vi "ER2007 Maintenance Panel.vi"() -> ()   [LabVIEW 2013]
uses:
  <vilib>/DAQmx/create/channels.llb/DAQmx Create Channel (DO-Digital Output).vi
  <vilib>/DAQmx/write.llb/DAQmx Write (Digital 1D Bool NChan 1Samp 1Line).vi
  Global ER2007.vi
  <vilib>/DAQmx/create/channels.llb/DAQmx Create Channel (DI-Digital Input).vi
  <vilib>/DAQmx/read.llb/DAQmx Read (Digital 1D Bool NChan 1Samp 1Line).vi
panel:
  out "Dev2Err":bool
  out "Lbl CJ1A":enum16{"CJ1A", "TC7B"}(ring)
  out "Lbl Pc1A":enum16{"Pc1A", "TC7A"}(ring)
  out "Lbl CJ1B":enum16{"CJ1B", "NOP8"}(ring)
  out "Lbl Pc1B":enum16{"Pc1B", "NOP7"}(ring)
  out "Lbl TC1B":enum16{"TC1B", "TC6B"}(ring)
  out "Lbl TC1A":enum16{"TC1A", "TC6A"}(ring)
  out "Lbl NOP1":enum16{"NOP1", "NOP6"}(ring)
  out "Ain 0-10":dbl format="%.3f"
  out "Ain 0-9":dbl format="%.3f"
  out "Ain 0-8":dbl format="%.3f"
  out "Ain 0-3":dbl format="%.3f"
  out "Ain 0-2":dbl format="%.3f"
  out "Ain 0-1":dbl format="%.3f"
  out "Ain 0-0":dbl format="%.3f"
  in  "Dout 1-0.11":bool
  in  "Dout 1-0.8":bool
  in  "Dout 1-0.13":bool
  out "Lbl PVol5":enum16{"PVol5", "PVol10"}(ring)
  out "Lbl PVol4":enum16{"PVol4", "PVol9"}(ring)
  out "Lbl PVol3":enum16{"PVol3", "PVol8"}(ring)
  out "Lbl PVol2":enum16{"PVol2", "PVol7"}(ring)
  out "Lbl PVol1":enum16{"PVol1", "PVol6"}(ring)
  out "Lbl Pdp5":enum16{"Pdp5", "Pdp10"}(ring)
  out "Lbl Pdp4":enum16{"Pdp4", "Pdp9"}(ring)
  out "Lbl Pdp3":enum16{"Pdp3", "Pdp8"}(ring)
  out "Lbl Pdp2":enum16{"Pdp2", "Pdp7"}(ring)
  out "Lbl Pdp1":enum16{"Pdp1", "Pdp6"}(ring)
  out "Lbl CJ5B":enum16{"CJ5B", "Pc10"}(ring)
  out "Lbl NOP5":enum16{"NOP5", "Pc9"}(ring)
  out "Lbl CJ3B":enum16{"CJ3B", "Pc8"}(ring)
  out "Lbl NOP3":enum16{"NOP3", "Pc7"}(ring)
  out "Lbl Pc2A":enum16{"Pc2A", "Pc6"}(ring)
  out "Lbl CJ5A":enum16{"CJ5A", "CJ9B"}(ring)
  out "Lbl Pc5B":enum16{"Pc5B", "CJ9A"}(ring)
  out "Lbl CJ4B":enum16{"CJ4B", "CJ8B"}(ring)
  out "Lbl CJ4A":enum16{"CJ4A", "CJ8A"}(ring)
  out "Lbl CJ3A":enum16{"CJ3A", "CJ7B"}(ring)
  out "Lbl Pc3B":enum16{"Pc3B", "CJ7A"}(ring)
  out "Lbl CJ2B":enum16{"CJ2B", "CJ6B"}(ring)
  out "Lbl CJ2A":enum16{"CJ2A", "CJ6A"}(ring)
  out "Lbl Pc4A":enum16{"Pc4A", "TC10B"}(ring)
  out "Lbl TC5B":enum16{"TC5B", "TC10A"}(ring)
  out "Lbl Pc5A":enum16{"Pc5A", "TC9B"}(ring)
  out "Lbl Pc4B":enum16{"Pc4B", "TC9A"}(ring)
  out "Lbl TC4A":enum16{"TC4A", "TC8B"}(ring)
  out "Lbl NOP4":enum16{"NOP4", "TC8A"}(ring)
  out "Lbl TC3A":enum16{"TC3A", "TC7B"}(ring)
  out "Lbl Pc3A":enum16{"Pc3A", "TC7A"}(ring)
  out "Lbl TC5A":enum16{"TC5A", "NOP10"}(ring)
  out "Lbl TC4B":enum16{"TC4B", "NOP9"}(ring)
  out "Lbl TC3B":enum16{"TC3B", "NOP8"}(ring)
  out "Lbl Pc2B":enum16{"Pc2B", "NOP7"}(ring)
  out "Lbl TC2B":enum16{"TC2B", "TC6B"}(ring)
  out "Lbl TC2A":enum16{"TC2A", "TC6A"}(ring)
  out "Lbl NOP2":enum16{"NOP2", "NOP6"}(ring)
  out "Ain 1-31":dbl format="%.3f"
  out "Ain 1-30":dbl format="%.3f"
  out "Ain 1-15":dbl format="%.3f"
  out "Ain 1-14":dbl format="%.3f"
  in  "Dout 1-0.3":bool
  in  "Dout 1-0.0":bool
  out "P0-2.1":bool caption="P2.1 - Busy 2"
  out "P0-2.0":bool caption="P2.0 - Busy 1"
  in  "Dout 0-1.6":bool
  out "Err 6":bool
  out "Err 5":bool
  out "NAII Time":u32
  out "NAII Err":i32
  in  "Wait (ms)":u32=1500
  out "Freq":dbl
  in  "Set":bool
  out "Err 3":bool
  out "Err 4":bool
  out "Exec Time":u32
  out "Signal":dbl format="%.4f"
  out "Phase":dbl format="%.3f"
  out "Reference":dbl format="%.4f"
  in  "Update":bool
  in  "Gen Off/On":bool
  in  "Ampl (Vrms)":dbl=1.0 min=0.1 max=10.0 format="%.2f"
  in  "Freq (Hz)":dbl=1000.0 min=20.0 max=100000.0
  out "Net 4-1":dbl format="%.3f"
  out "Net 4-0":dbl format="%.3f"
  out "Net 3-1":dbl format="%.3f"
  out "Net 3-0":dbl format="%.3f"
  out "Net 2-1":dbl format="%.3f"
  out "Net 2-0":dbl format="%.3f"
  out "Net 1-1":dbl format="%.3f"
  out "Net 1-0":dbl format="%.3f"
  out "Net 0-1":dbl format="%.3f"
  out "Net 0-0":dbl format="%.3f"
  in  "EUs 1":bool
  out "Ain 1-29":dbl format="%.3f"
  out "Ain 1-27":dbl format="%.3f"
  out "Ain 1-26":dbl format="%.3f"
  out "Ain 1-25":dbl format="%.3f"
  out "Ain 1-24":dbl format="%.3f"
  out "Ain 1-23":dbl format="%.3f"
  out "Ain 1-22":dbl format="%.3f"
  out "Ain 1-21":dbl format="%.3f"
  out "Ain 1-19":dbl format="%.3f"
  out "Ain 1-18":dbl format="%.3f"
  out "Ain 1-17":dbl format="%.3f"
  out "Ain 1-16":dbl format="%.3f"
  in  "EUs 0":bool
  out "Ain 1-13":dbl format="%.3f"
  out "Ain 1-11":dbl format="%.3f"
  out "Ain 1-10":dbl format="%.3f"
  out "Ain 1-9":dbl format="%.3f"
  out "Ain 1-8":dbl format="%.3f"
  out "Ain 1-7":dbl format="%.3f"
  out "Ain 1-6":dbl format="%.3f"
  out "Ain 1-5":dbl format="%.3f"
  out "Ain 1-3":dbl format="%.3f"
  out "Ain 1-2":dbl format="%.3f"
  out "Ain 1-1":dbl format="%.3f"
  out "Ain 1-0":dbl format="%.3f"
  out "Err 7":bool
  in  "AllOff 0":bool
  in  "Dout 0-1.4":bool
  in  "Dout 0-1.3":bool
  in  "Dout 0-1.2":bool
  in  "Dout 0-1.1":bool
  in  "Dout 0-1.0":bool
  in  "Dout 0-0.7":bool
  in  "Dout 1-0.5":bool
  in  "Dout 0-0.5":bool
  in  "Dout 0-0.4":bool
  in  "Dout 0-0.3":bool
  out "Dev1Err":bool
  in  "Dout 0-0.2":bool
  in  "Dout 0-0.1":bool
  in  "Dout 0-0.0":bool
  in  "Exit":bool
  # "ER2007 Maintenance Panel"
  # "Galil CDS-3310"
  # "Dev1 PCI-6220 Douts"
  # "Dev1 PCI-6220 Ains"
  # "Dev2 PCI-6224 Analog Ins"
  # "GPIB0 - Signal Gen"
  # "Error"
  # "Dev2 PCI-6224 Douts"
  # "PCI-6224 Dins"
  # "Error"
  # "GPIB1 - Volts/Phase"
  # "Error"
  # "Error"
  # "Error"
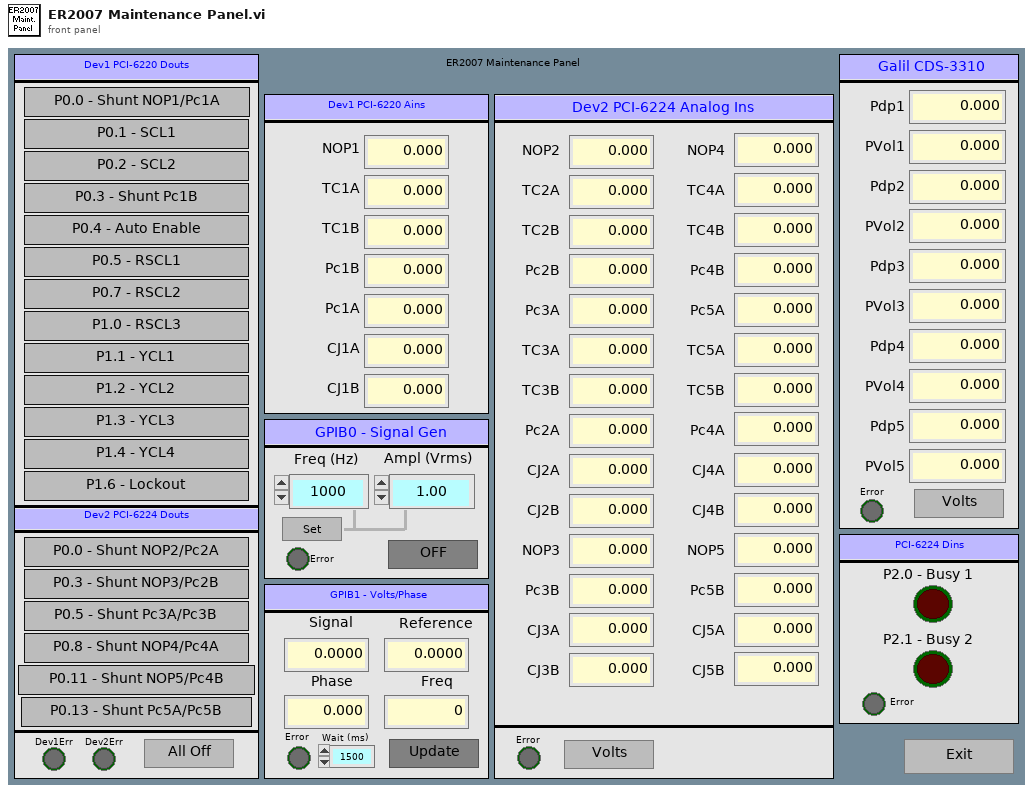
[diagram p1: front panel]
types:
  T1 = enum16{"TOTAL", "FUNDAMENTAL", "IN PHASE", "QUADRATURE", "PHASE ANGLE", "THD"}
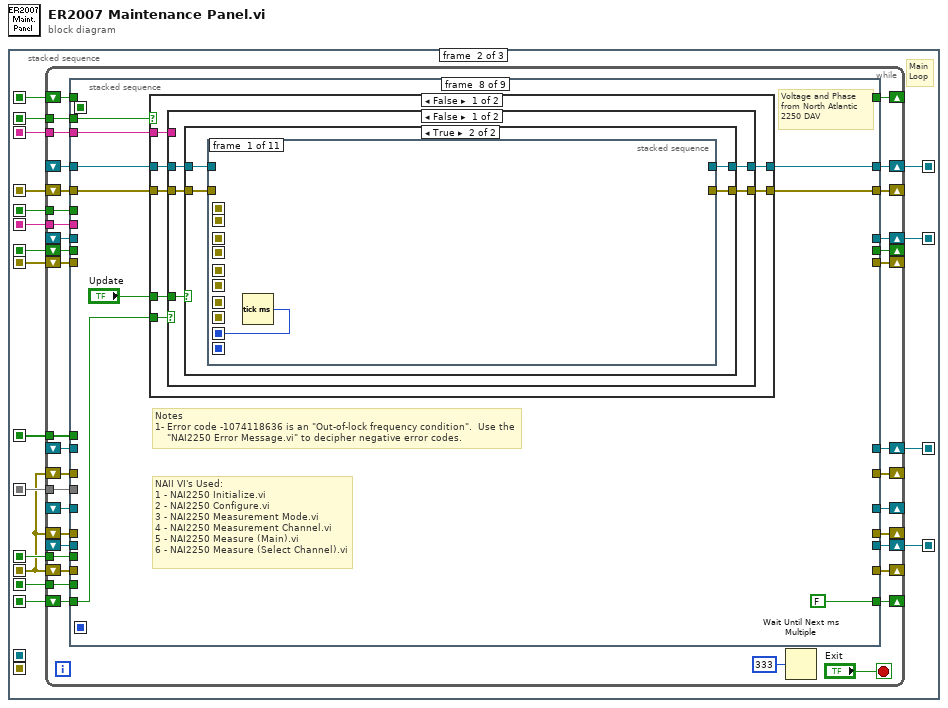
[diagram p0: block diagram]
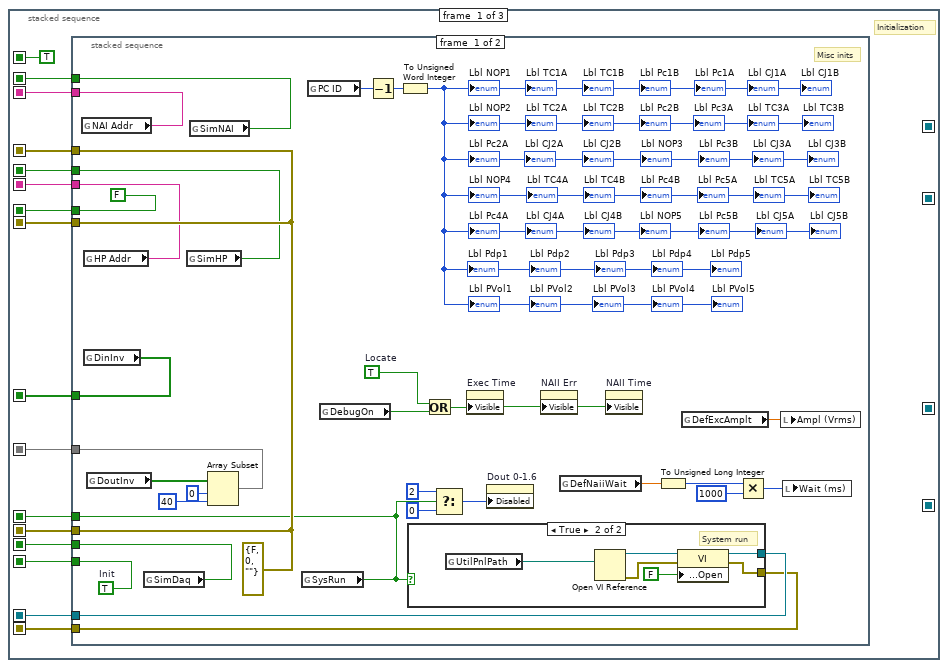
[diagram p2: hidden frame]
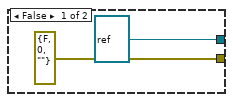
[diagram p3: hidden frame]
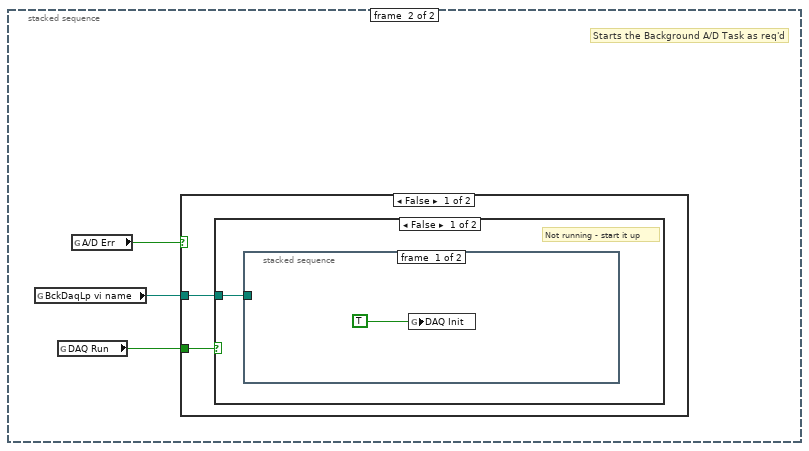
[diagram p4: hidden frame]
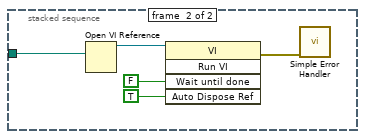
[diagram p5: hidden frame]
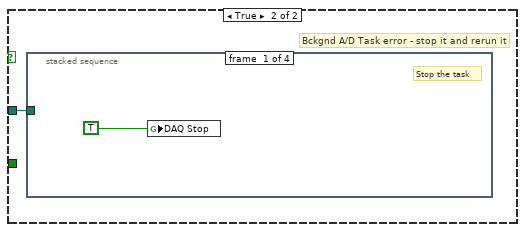
[diagram p7: hidden frame]
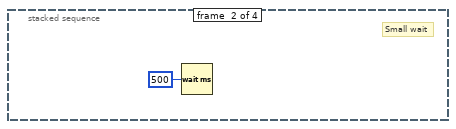
[diagram p8: hidden frame]
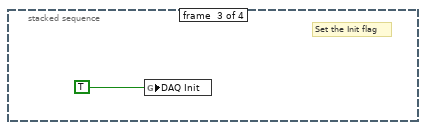
[diagram p9: hidden frame]
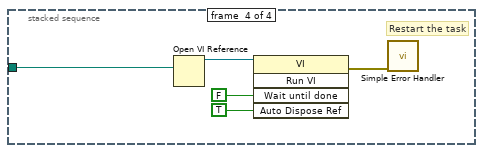
[diagram p10: hidden frame]
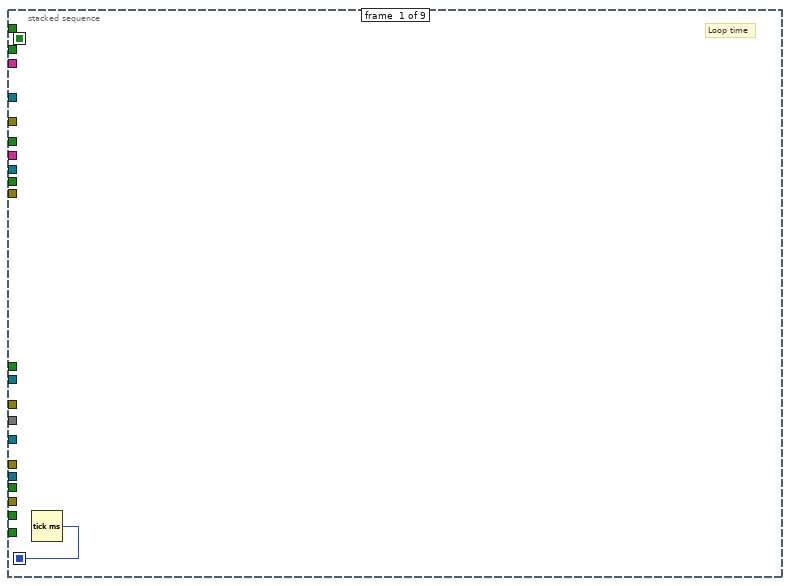
[diagram p11: hidden frame]
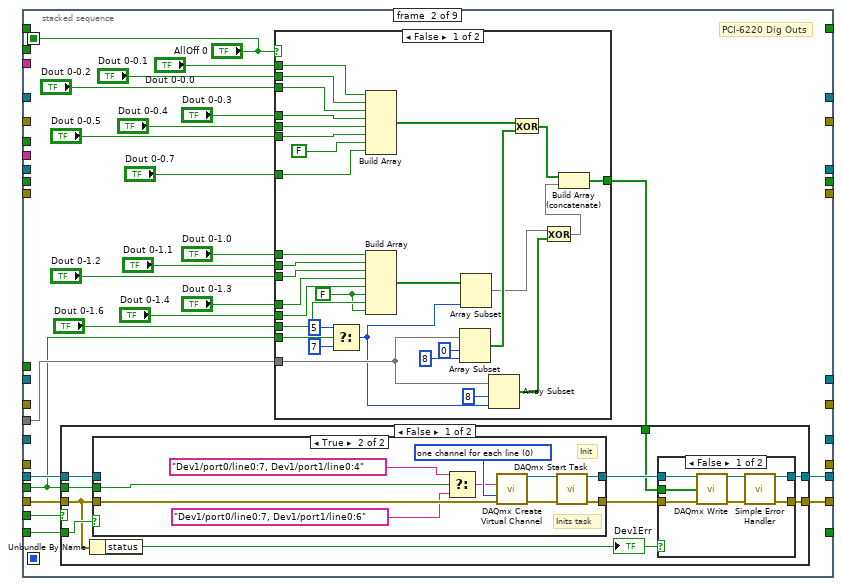
[diagram p12: hidden frame]
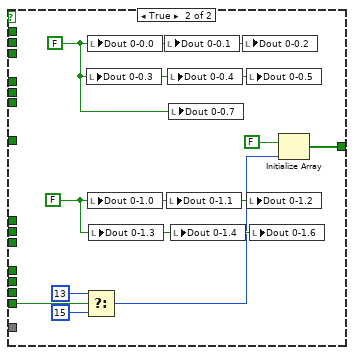
[diagram p16: hidden frame]
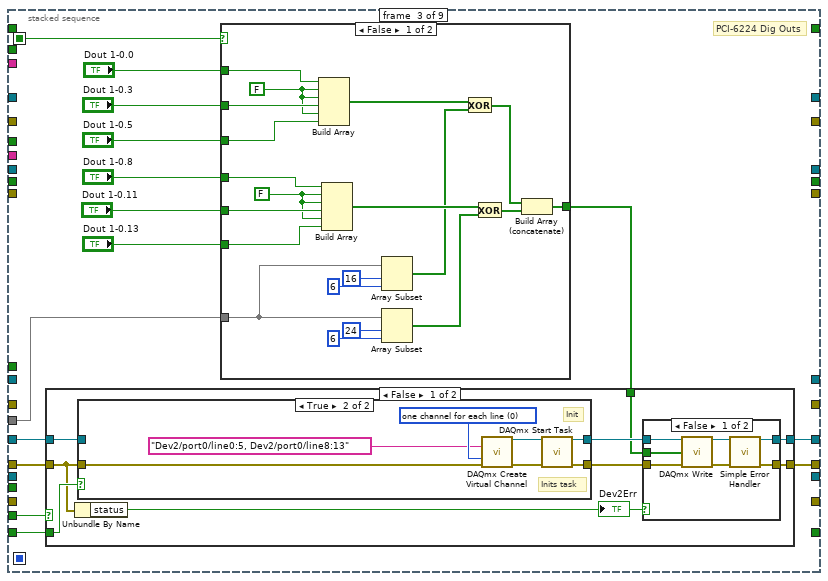
[diagram p17: hidden frame]
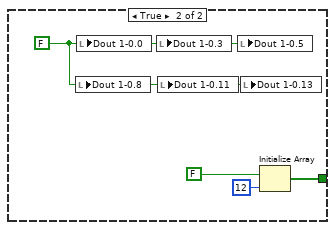
[diagram p18: hidden frame]
diagram:
  n1 = stacked-sequence {
    seq-local: [w16 _ _] -> [_ w91 _]
    seq-local: [w15 _ _] -> [_ w93 _]
    seq-local: [w14 _ _] -> [_ w76 _]
    seq-local: [w13 _ _] -> [_ w92 w633]
    seq-local: [w12 _ _] -> [_ w78 w638]
    seq-local: [w11 _ _] -> [_ _ w640]
    seq-local: [w10 _ _] -> [_ _ w639]
    seq-local: [_ w90 _] -> [_ _ w637]
    seq-local: [_ w89 _] -> [_ _ w636]
    seq-local: [w9 _ _] -> [_ w88 w632]
    seq-local: [w8 _ _] -> [_ w86 _]
    seq-local: [w7 _ _] -> [_ w87 _]
    seq-local: [w6 _ _] -> [_ w85 w631]
    seq-local: [w5 _ _] -> [_ w84 _]
    seq-local: [w4 _ _] -> [_ w83 _]
    seq-local: [w3 _ _] -> [_ w82 _]
    seq-local: [_ w81 _] -> [_ _ w635]
    seq-local: [_ w80 _] -> [_ _ w634]
    seq-local: [w2 _ _] -> [_ w79 _]
    seq-local: [TRUE _ _] -> [_ w77 _]
    frame #0 {
      # "Initialization"
      n2 = stacked-sequence {
        tunnel: [w29 _] -> w16
        tunnel: [w46 _] -> w15
        tunnel: [w43 _] -> w14
        tunnel: [w35 _] -> w13
        tunnel: [w25 _] -> w12
        tunnel: [w45 _] -> w11
        tunnel: [w44 _] -> w10
        tunnel: [w41 _] -> w9
        tunnel: [w40 _] -> w8
        tunnel: [w43 _] -> w7
        tunnel: [w38 _] -> w6
        tunnel: [w39 _] -> w5
        tunnel: [w43 _] -> w4
        tunnel: [FALSE _] -> w3
        tunnel: [w34 _] -> w2
        frame #0 {
          w26 = TRUE  # Locate
          w43 = errorcluster {"status"=FALSE, "code"=0, "source"=""} ("error out")
          w46 = TRUE  # Init
          # "Misc inits"
          n3 = global read "Global ER2007.vi" "NAI Addr"() -> (w40:string)
          n4 = global read "Global ER2007.vi" "HP Addr"() -> (w39:string)
          n5 = global read "Global ER2007.vi" "DinInv"() -> (w34:bool[])
          n6 = global read "Global ER2007.vi" "DoutInv"() -> (w30:bool[])
          n7 = global read "Global ER2007.vi" "SimDaq"() -> (w35:bool)
          n8 = global read "Global ER2007.vi" "SimHP"() -> (w38:bool)
          n9 = global read "Global ER2007.vi" "SimNAI"() -> (w41:bool)
          n10 = Array Subset(array=w30, index=0, length=40) -> (w29:bool[])
          n11 = global read "Global ER2007.vi" "SysRun"() -> (w25:bool)
          n12 = global read "Global ER2007.vi" "PC ID"() -> (w21:i32)
          n13 = global read "Global ER2007.vi" "DebugOn"() -> (w28:bool)
          n14 = Decrement(x=w21) -> (x-1=w20:i32)
          n15 = To Unsigned Word Integer(number=w20) -> (unsigned 16bit integer=→"Lbl NOP2" →"Lbl TC2A" →"Lbl Pc2A" →"Lbl TC4B" →"Lbl TC5A" →"Lbl CJ5B" →"Lbl NOP5" →"Lbl CJ3B" →"Lbl CJ5A" →"Lbl Pc4A" →"Lbl Pc5A" →"Lbl Pc2B" →"Lbl TC3B" →"Lbl TC3A" →"Lbl TC4A" →"Lbl CJ2B" →"Lbl CJ3A" →"Lbl CJ4B" →"Lbl NOP3" →"Lbl CJ4A" →"Lbl CJ2A" →"Lbl Pc3A" →"Lbl NOP4" →"Lbl Pc3B" →"Lbl Pc4B" →"Lbl Pc5B" →"Lbl TC2B" →"Lbl TC5B" →"Lbl Pdp1" →"Lbl Pdp2" →"Lbl Pdp3" →"Lbl Pdp4" →"Lbl Pdp5" →"Lbl PVol1" →"Lbl PVol2" →"Lbl PVol3" →"Lbl PVol4" →"Lbl PVol5" →"Lbl NOP1" →"Lbl TC1A" →"Lbl TC1B" →"Lbl Pc1B" →"Lbl Pc1A" →"Lbl CJ1A" →"Lbl CJ1B":u16)
          n16 = case shown="True" w25 {
            tunnel: [refnum<vi> refnum w51] -> w45
            tunnel: [errorcluster {"status"=FALSE, "code"=0, "source"=""} ("error out") w50] -> w44
            frame False {
            }
            frame True {
              # "System run"
              n17 = global read "Global ER2007.vi" "UtilPnlPath"() -> (w49:path)
              n18 = Open VI Reference(vi path=w49) -> (vi reference=w54:refnum<vi>, error out=w53:errorcluster)  [unwired: 5 in]
              n19 = property class="VI"(reference=w54, error in=w53, "Front Panel Window:Open"=FALSE) -> (reference out=w51:refnum<vi>, error out=w50:errorcluster)
            }
          }
          n20 = Or(x=w26, y=w28) -> (x .or. y?=w27:bool)
          n21 = Select(t=u8 2, s=w25, f=u8 0 ("Disabled")) -> (s? t:f=w24:u8)
          n22 = property on="Exec Time" class="DigNum (strict)"("Visible"=w27) -> ()  [unwired: 2 in, 2 out]
          n23 = property on="Dout 0-1.6" class="Bool (strict)"("Disabled"=w24) -> ()  [unwired: 2 in, 2 out]
          n24 = property on="NAII Err" class="DigNum (strict)"("Visible"=w27) -> ()  [unwired: 2 in, 2 out]
          n25 = global read "Global ER2007.vi" "DefNaiiWait"() -> (w36:dbl)
          n26 = property on="NAII Time" class="DigNum (strict)"("Visible"=w27) -> ()  [unwired: 2 in, 2 out]
          n27 = To Unsigned Long Integer(number=w36) -> (unsigned 32bit integer=w33:u32)
          n28 = global read "Global ER2007.vi" "DefExcAmplt"() -> (w37:dbl)
          n29 = Multiply(x=w33, y=u32 1000) -> (x*y=w18:u32)
          n30 = local write "Ampl (Vrms)"(w37) -> ()
          n31 = local write "Wait (ms)"(w18) -> ()
        }
        frame #1 {
          # "Starts the Background A/D Task as req'd"
          n32 = global read "Global ER2007.vi" "BckDaqLp vi name"() -> (w56:path)
          n33 = global read "Global ER2007.vi" "DAQ Run"() -> (w55:bool)
          n34 = global read "Global ER2007.vi" "A/D Err"() -> (w57:bool)
          n35 = case shown="False" w57 {
            tunnel: w55 -> [w59 _]
            tunnel: w56 -> [w58 w67]
            frame False {
              n36 = case shown="False" w59 {
                tunnel: w58 -> [w60 _]
                frame False {
                  # "Not running - start it up"
                  n37 = stacked-sequence {
                    tunnel: w60 -> [_ w62]
                    frame #0 {
                      n38 = global write "Global ER2007.vi" "DAQ Init"(TRUE ("A/D Init")) -> ()
                    }
                    frame #1 {
                      n39 = Open VI Reference(vi path=w62) -> (vi reference=w66:refnum<vi>)  [unwired: 5 in, 1 out]
                      n40 = invoke class="VI" method="Run VI"(reference=w66, "Wait until done"=FALSE, "Auto Dispose Ref"=TRUE) -> (error out=w63:errorcluster)  [unwired: 2 in, 4 out]
                      n41 = call <vilib>:"Simple Error Handler.vi"("error in (no error)"=w63) -> ()  [unwired: 4 in, 5 out]
                    }
                  }
                }
                frame True {
                  # "The bckgnd task is already\nrunning - do nothing"
                }
              }
            }
            frame True {
              # "Bckgnd A/D Task error - stop it and rerun it"
              n42 = stacked-sequence {
                tunnel: w67 -> [_ _ _ w71]
                frame #0 {
                  # "Stop the task"
                  n43 = global write "Global ER2007.vi" "DAQ Stop"(TRUE ("A/D Stop")) -> ()
                }
                frame #1 {
                  # "Small wait"
                  n44 = Wait (ms)(milliseconds to wait=u32 500) -> ()  [unwired: 1 out]
                }
                frame #2 {
                  # "Set the Init flag"
                  n45 = global write "Global ER2007.vi" "DAQ Init"(TRUE ("A/D Init")) -> ()
                }
                frame #3 {
                  # "Restart the task"
                  n46 = Open VI Reference(vi path=w71) -> (vi reference=w75:refnum<vi>)  [unwired: 5 in, 1 out]
                  n47 = invoke class="VI" method="Run VI"(reference=w75, "Wait until done"=FALSE, "Auto Dispose Ref"=TRUE) -> (error out=w72:errorcluster)  [unwired: 2 in, 4 out]
                  n48 = call <vilib>:"Simple Error Handler.vi"("error in (no error)"=w72) -> ()  [unwired: 4 in, 5 out]
                }
              }
            }
          }
        }
      }
    }
    frame #1 {
      # "Main\nLoop"
      n49 = while {
        shift-right: [w127] -> _
        shift-left: w93 -> [w126]
        shift-right: [w124] -> _
        shift-left: w76 -> [w125]
        shift-right: [w123] -> w90
        shift-left: _ -> [w122]
        tunnel: w92 -> [w121]
        tunnel: w91 -> [w120]
        shift-right: [w116] -> _
        shift-left: w76 -> [w119]
        shift-right: [w117] -> w89
        shift-left: _ -> [w118]
        tunnel: w88 -> [w115]
        shift-right: [w113] -> _
        shift-left: w87 -> [w114]
        tunnel: w86 -> [w112]
        shift-right: [w111] -> w80
        shift-left: _ -> [w110]
        tunnel: w85 -> [w109]
        tunnel: w84 -> [w108]
        shift-right: [w106] -> _
        shift-left: w83 -> [w107]
        shift-right: [w105] -> w81
        shift-left: _ -> [w104]
        shift-right: [w102] -> _
        shift-left: w82 -> [w103]
        tunnel: w79 -> [w101]
        tunnel: w78 -> [w100]
        shift-right: [w99] -> _
        shift-left: w77 -> [w98]
        shift-right: [w95] -> _
        shift-left: _ -> [w96]
        shift-right: [w94] -> _
        shift-left: w76 -> [w97]
        stop <- "Exit" stop-if-true
        n50 = stacked-sequence {
          seq-local: [w130 _ _ _ _ _ _ _ _] -> [_ _ _ _ _ _ _ _ w629]
          seq-local: [_ "AllOff 0" _ _ _ _ _ _ _] -> [_ _ w233 _ _ _ _ _ _]
          tunnel: [_ _ _ _ _ _ _ FALSE _] -> w127
          tunnel: w126 -> [_ w153 w235 w304 _ _ w427 w485 _]
          tunnel: w125 -> [_ w152 _ _ _ _ _ _ _]
          tunnel: [_ w151 _ _ _ _ _ _ _] -> w124
          tunnel: [_ w150 _ _ _ _ _ _ _] -> w123
          tunnel: w122 -> [_ w149 _ _ _ _ _ _ _]
          tunnel: w121 -> [_ w135 w234 w305 _ _ _ _ _]
          tunnel: w120 -> [_ w134 w225 _ _ _ _ _ _]
          tunnel: w119 -> [_ _ _ w303 _ _ _ _ _]
          tunnel: w118 -> [_ _ _ w302 _ _ _ _ _]
          tunnel: [_ _ _ w301 _ _ _ _ _] -> w117
          tunnel: [_ _ _ w300 _ _ _ _ _] -> w116
          tunnel: w115 -> [_ _ _ _ _ _ _ w488 _]
          tunnel: w114 -> [_ _ _ _ _ _ _ w487 _]
          tunnel: [_ _ _ _ _ _ _ w486 _] -> w113
          tunnel: w112 -> [_ _ _ _ _ _ _ w484 _]
          tunnel: [_ _ _ _ _ _ _ w483 _] -> w111
          tunnel: w110 -> [_ _ _ _ _ _ _ w482 _]
          tunnel: w109 -> [_ _ _ _ _ _ w429 _ _]
          tunnel: w108 -> [_ _ _ _ _ _ w428 _ _]
          tunnel: w107 -> [_ _ _ _ _ _ w426 _ _]
          tunnel: [_ _ _ _ _ _ w425 _ _] -> w106
          tunnel: [_ _ _ _ _ _ w424 _ _] -> w105
          tunnel: w104 -> [_ _ _ _ _ _ w423 _ _]
          tunnel: w103 -> [_ _ _ _ _ _ w422 _ _]
          tunnel: [_ _ _ _ _ _ w421 _ _] -> w102
          tunnel: w101 -> [_ _ _ w294 _ _ _ _ _]
          tunnel: w100 -> [_ w132 _ w293 _ _ _ _ _]
          tunnel: [_ _ _ _ "EUs 0" _ _ _ _] -> w99
          tunnel: w98 -> [_ _ _ _ w388 _ _ _ _]
          tunnel: w97 -> [_ _ w239 _ _ _ _ _ _]
          tunnel: w96 -> [_ _ w238 _ _ _ _ _ _]
          tunnel: [_ _ w237 _ _ _ _ _ _] -> w95
          tunnel: [_ _ w236 _ _ _ _ _ _] -> w94
          frame #0 {
            # "Loop time"
            n51 = Tick Count (ms)() -> (millisecond timer value=w130:u32)
          }
          frame #1 {
            # "PCI-6220 Dig Outs"
            n52 = case shown="False" "AllOff 0" {
              tunnel: "Dout 0-0.0" -> [w216 _]
              tunnel: "Dout 0-0.1" -> [w215 _]
              tunnel: "Dout 0-0.2" -> [w214 _]
              tunnel: "Dout 0-0.3" -> [w213 _]
              tunnel: "Dout 0-0.4" -> [w212 _]
              tunnel: "Dout 0-0.5" -> [w211 _]
              tunnel: "Dout 0-0.7" -> [w210 _]
              tunnel: "Dout 0-1.0" -> [w203 _]
              tunnel: "Dout 0-1.1" -> [w204 _]
              tunnel: "Dout 0-1.2" -> [w205 _]
              tunnel: "Dout 0-1.3" -> [w202 _]
              tunnel: "Dout 0-1.4" -> [w201 _]
              tunnel: [w198 w223] -> w136
              tunnel: w134 -> [w195 _]
              tunnel: "Dout 0-1.6" -> [w197 _]
              tunnel: w132 -> [w188 w220]
              frame False {
                w196 = FALSE ("element")
                n53 = Select(t=5 ("length"), s=w188, f=7) -> (s? t:f=w187:i32)
                n54 = Build Array(w216, w215, w214, w213, w212, w211, FALSE ("element"), w210) -> (w209:bool[])
                n55 = Build Array(w203, w204, w205, w202, w201, w196, w197, w196) -> (w194:bool[])
                n56 = Array Subset(array=w195, index=0, length=8) -> (w206:bool[])
                n57 = Array Subset(array=w194, length=w187) -> (w193:bool[])  [unwired: 1 in]
                n58 = Array Subset(array=w195, index=8, length=w187) -> (w200:bool[])
                n59 = Exclusive Or(1:w206, 2:w209) -> (0:w199:bool[])
                n60 = Exclusive Or(1:w200, 2:w193) -> (0:w191:bool[])
                n61 = Build Array (concatenate)(w199, w191) -> (w198:bool[])
              }
              frame True {
                w221 = FALSE ("Dout 0-1.0")
                w222 = FALSE ("Dout 0-0.1")
                n62 = Select(t=13 ("dimension size"), s=w220, f=15 ("dimension size")) -> (s? t:f=w217:i32)
                n63 = local write "Dout 0-0.3"(w222) -> ()
                n64 = local write "Dout 0-0.0"(w222) -> ()
                n65 = local write "Dout 0-1.0"(w221) -> ()
                n66 = local write "Dout 0-1.3"(w221) -> ()
                n67 = local write "Dout 0-0.1"(w222) -> ()
                n68 = local write "Dout 0-1.1"(w221) -> ()
                n69 = local write "Dout 0-0.4"(w222) -> ()
                n70 = local write "Dout 0-0.7"(w222) -> ()
                n71 = local write "Dout 0-1.4"(w221) -> ()
                n72 = local write "Dout 0-0.2"(w222) -> ()
                n73 = local write "Dout 0-0.5"(w222) -> ()
                n74 = local write "Dout 0-1.2"(w221) -> ()
                n75 = local write "Dout 0-1.6"(w221) -> ()
                n76 = Initialize Array(FALSE, w217) -> (w223:bool[])
              }
            }
            n77 = case shown="False" w135 {
              tunnel: w153 -> [w163 _]
              tunnel: w152 -> [w156 w184]
              tunnel: [w161 w184] -> w151
              tunnel: [w160 w185] -> w150
              tunnel: w149 -> [w158 w185]
              tunnel: w136 -> [w157 _]
              tunnel: w132 -> [w154 _]
              frame False {
                n78 = Unbundle By Name(w156) -> ("status"=w155:bool)
                "Dev1Err" <- w155
                n79 = case shown="True" w163 {
                  tunnel: w156 -> [w172 w181]
                  tunnel: [w173 w180] -> w162
                  tunnel: [w172 w179] -> w159
                  tunnel: w158 -> [w173 _]
                  tunnel: w154 -> [_ w174]
                  frame False {
                  }
                  frame True {
                    w178 = 0 items=["one channel for each line", "one channel for all lines"] ("line grouping")
                    # "Init"
                    # "Inits task"
                    n80 = Select(t=tag "Dev1/port0/line0:7, Dev1/port1/line0:4" ("lines"), s=w174, f=tag "Dev1/port0/line0:7, Dev1/port1/line0:6" ("lines")) -> (s? t:f=w177:tag)
                    n81 = call-poly <vilib>:"DAQmx Create Virtual Channel.vi"("lines"=w177, "line grouping"=w178, "error in"=w181) -> ("task out"=w183:refnum<k21>, "error out"=w182:errorcluster)  [unwired: 11 in]
                    n82 = call <vilib>:"DAQmx Start Task.vi"("task/channels in"=w183, "error in"=w182) -> ("task out"=w180:refnum<k21>, "error out"=w179:errorcluster)  [unwired: 12 in]
                  }
                }
                n83 = case shown="False" w155 {
                  tunnel: w159 -> [w169 w170]
                  tunnel: w162 -> [w168 w171]
                  tunnel: [w165 w170] -> w161
                  tunnel: [w167 w171] -> w160
                  tunnel: w157 -> [w164 _]
                  frame False {
                    n84 = call-poly <vilib>:"DAQmx Write.vi"("task/channels in"=w168, "data"=w164, "error in"=w169) -> ("task out"=w167:refnum<k21>, "error out"=w166:errorcluster)  [unwired: 10 in, 1 out]
                    n85 = call <vilib>:"Simple Error Handler.vi"("error in (no error)"=w166) -> ("error out"=w165:errorcluster)  [unwired: 4 in, 4 out]
                  }
                  frame True {
                    # "Prev error"
                  }
                }
              }
              frame True {
                # "Simulation"
              }
            }
          }
          frame #2 {
            # "PCI-6224 Dig Outs"
            n86 = case shown="False" w233 {
              tunnel: "Dout 1-0.3" -> [w259 _]
              tunnel: "Dout 1-0.0" -> [w258 _]
              tunnel: "Dout 1-0.5" -> [w257 _]
              tunnel: "Dout 1-0.11" -> [w255 _]
              tunnel: "Dout 1-0.8" -> [w254 _]
              tunnel: "Dout 1-0.13" -> [w253 _]
              tunnel: [w251 w261] -> w226
              tunnel: w225 -> [w241 _]
              frame False {
                w252 = FALSE ("element")
                w256 = FALSE ("element")
                n87 = Build Array(w258, w256, w256, w259, w256, w257) -> (w250:bool[])
                n88 = Build Array(w254, w252, w252, w255, w252, w253) -> (w249:bool[])
                n89 = Array Subset(array=w241, index=16, length=6) -> (w244:bool[])
                n90 = Array Subset(array=w241, index=24, length=6) -> (w240:bool[])
                n91 = Exclusive Or(1:w244, 2:w250) -> (0:w247:bool[])
                n92 = Exclusive Or(1:w240, 2:w249) -> (0:w248:bool[])
                n93 = Build Array (concatenate)(w247, w248) -> (w251:bool[])
              }
              frame True {
                w263 = FALSE
                n94 = local write "Dout 1-0.8"(w263) -> ()
                n95 = local write "Dout 1-0.0"(w263) -> ()
                n96 = local write "Dout 1-0.3"(w263) -> ()
                n97 = local write "Dout 1-0.11"(w263) -> ()
                n98 = local write "Dout 1-0.5"(w263) -> ()
                n99 = local write "Dout 1-0.13"(w263) -> ()
                n100 = Initialize Array(FALSE, 12 ("dimension size")) -> (w261:bool[])
              }
            }
            n101 = case shown="False" w234 {
              tunnel: w235 -> [w272 _]
              tunnel: w239 -> [w265 w290]
              tunnel: [w270 w290] -> w236
              tunnel: [w269 w291] -> w237
              tunnel: w238 -> [w267 w291]
              tunnel: w226 -> [w266 _]
              frame False {
                n102 = Unbundle By Name(w265) -> ("status"=w264:bool)
                "Dev2Err" <- w264
                n103 = case shown="True" w272 {
                  tunnel: w265 -> [w281 w287]
                  tunnel: [w282 w286] -> w271
                  tunnel: [w281 w285] -> w268
                  tunnel: w267 -> [w282 _]
                  frame False {
                  }
                  frame True {
                    w284 = 0 items=["one channel for each line", "one channel for all lines"] ("line grouping")
                    # "Init"
                    # "Inits task"
                    n104 = call-poly <vilib>:"DAQmx Create Virtual Channel.vi"("lines"=tag "Dev2/port0/line0:5, Dev2/port0/line8:13", "line grouping"=w284, "error in"=w287) -> ("task out"=w289:refnum<k21>, "error out"=w288:errorcluster)  [unwired: 11 in]
                    n105 = call <vilib>:"DAQmx Start Task.vi"("task/channels in"=w289, "error in"=w288) -> ("task out"=w286:refnum<k21>, "error out"=w285:errorcluster)  [unwired: 12 in]
                  }
                }
                n106 = case shown="False" w264 {
                  tunnel: w268 -> [w278 w279]
                  tunnel: w271 -> [w277 w280]
                  tunnel: [w274 w279] -> w270
                  tunnel: [w276 w280] -> w269
                  tunnel: w266 -> [w273 _]
                  frame False {
                    n107 = call-poly <vilib>:"DAQmx Write.vi"("task/channels in"=w277, "data"=w273, "error in"=w278) -> ("task out"=w276:refnum<k21>, "error out"=w275:errorcluster)  [unwired: 10 in, 1 out]
                    n108 = call <vilib>:"Simple Error Handler.vi"("error in (no error)"=w275) -> ("error out"=w274:errorcluster)  [unwired: 4 in, 4 out]
                  }
                  frame True {
                    # "Prev error"
                  }
                }
              }
              frame True {
                # "Simulation"
              }
            }
          }
          frame #3 {
            w297 = 1  # Busy 2
            w298 = 0  # Busy 1
            # "PCI-6224 Dig Ins"
            n109 = case shown="False" w305 {
              tunnel: w304 -> [w313 _]
              tunnel: w303 -> [w309 w349]
              tunnel: [w312 w349] -> w300
              tunnel: [w310 w350] -> w301
              tunnel: w302 -> [w306 w350]
              tunnel: [w308 bool[] [FALSE, FALSE] ("data")] -> w292
              tunnel: w293 -> [w311 _]
              frame False {
                n110 = Unbundle By Name(w309) -> ("status"=→"Err 7":bool)
                n111 = global read "Global ER2007.vi" "BoxBusy"() -> (w307:bool[])
                n112 = case shown="True" w313 {
                  tunnel: [w315 w335] -> w312
                  tunnel: w311 -> [w321 w334]
                  tunnel: [w316 w333] -> w310
                  tunnel: w309 -> [w320 w332]
                  tunnel: [w318 w331] -> w308
                  tunnel: w307 -> [w317 w330]
                  tunnel: w306 -> [w319 _]
                  frame False {
                    n113 = case shown="False" w321 {
                      tunnel: w320 -> [w325 w327]
                      tunnel: w319 -> [w326 w328]
                      tunnel: [w322 w329] -> w318
                      tunnel: w317 -> [_ w329]
                      tunnel: [w323 w328] -> w316
                      tunnel: [w324 w327] -> w315
                      frame False {
                        # "NOT a SysRun - real I/O"
                        n114 = call-poly <vilib>:"DAQmx Read.vi"("task/channels in"=w326, "error in"=w325) -> ("task out"=w323:refnum<k21>, "data"=w322:bool[], "error out"=w324:errorcluster)  [unwired: 11 in]
                      }
                      frame True {
                        # "System Run - can't do real I/O here"
                      }
                    }
                  }
                  frame True {
                    # "Init"
                    n115 = case shown="False" w334 {
                      tunnel: [w339 errorcluster {"status"=FALSE, "code"=0, "source"=""} ("error out")] -> w335
                      tunnel: [w338 refnum<k21> refnum ("task out")] -> w333
                      tunnel: w332 -> [_ _]
                      tunnel: [w337 w346] -> w331
                      tunnel: w330 -> [_ w346]
                      frame False {
                        w344 = 0 items=["one channel for each line", "one channel for all lines"] ("line grouping")
                        # "NOT a SysRun - real I/O"
                        n116 = call-poly <vilib>:"DAQmx Create Virtual Channel.vi"("lines"=tag "Dev1/port2/line0:1", "line grouping"=w344) -> ("task out"=w342:refnum<k21>, "error out"=w343:errorcluster)  [unwired: 12 in]
                        n117 = call <vilib>:"DAQmx Start Task.vi"("task/channels in"=w342, "error in"=w343) -> ("task out"=w341:refnum<k21>, "error out"=w340:errorcluster)  [unwired: 12 in]
                        n118 = call-poly <vilib>:"DAQmx Read.vi"("task/channels in"=w341, "error in"=w340) -> ("task out"=w338:refnum<k21>, "data"=w337:bool[], "error out"=w339:errorcluster)  [unwired: 11 in]
                      }
                      frame True {
                        # "System Run - can't do real I/O here"
                      }
                    }
                  }
                }
              }
              frame True {
                # "Simulation"
              }
            }
            n119 = Exclusive Or(1:w292, 2:w294) -> (0:w295:bool[])
            n120 = Index Array(array=w295, index #1=w298, index #2=w297) -> (element #1=→"P0-2.0":bool, element #2=→"P0-2.1":bool)
          }
          frame #4 {
            # "PCI-6224 AINs"
            n121 = Not Equal?(x=w388, y="EUs 0") -> (x != y?=w387:bool)
            n122 = case shown="True" w387 {
              tunnel: "EUs 0" -> [_ w395]
              frame False {
              }
              frame True {
                n123 = Select(t=u8 0 ("Format & Precision:Precision"), s=w395, f=u8 3 ("Format & Precision:Precision")) -> (s? t:f=w394:u8)
                n124 = Select(t=u8 0 ("Format & Precision:Precision"), s=w395, f=u8 3 ("Format & Precision:Precision")) -> (s? t:f=w398:u8)
                n125 = property on="Ain 1-8" class="DigNum (strict)"("Display Format:Precision"=w394) -> ()  [unwired: 2 in, 2 out]
                n126 = property on="Ain 1-0" class="DigNum (strict)"("Display Format:Precision"=w398) -> ()  [unwired: 2 in, 2 out]
                n127 = property on="Ain 1-3" class="DigNum (strict)"("Display Format:Precision"=w398) -> ()  [unwired: 2 in, 2 out]
                n128 = property on="Ain 1-11" class="DigNum (strict)"("Display Format:Precision"=w394) -> ()  [unwired: 2 in, 2 out]
                n129 = property on="Ain 1-7" class="DigNum (strict)"("Display Format:Precision"=w398) -> ()  [unwired: 2 in, 2 out]
                n130 = property on="Ain 1-15" class="DigNum (strict)"("Display Format:Precision"=w394) -> ()  [unwired: 2 in, 2 out]
                n131 = property on="Ain 1-18" class="DigNum (strict)"("Display Format:Precision"=w398) -> ()  [unwired: 2 in, 2 out]
                n132 = property on="Ain 1-27" class="DigNum (strict)"("Display Format:Precision"=w394) -> ()  [unwired: 2 in, 2 out]
                n133 = property on="Ain 1-22" class="DigNum (strict)"("Display Format:Precision"=w398) -> ()  [unwired: 2 in, 2 out]
                n134 = property on="Ain 1-31" class="DigNum (strict)"("Display Format:Precision"=w394) -> ()  [unwired: 2 in, 2 out]
              }
            }
            n135 = case shown="False" "EUs 0" {
              tunnel: [w401 w402] -> w391
              frame False {
                # "Volts"
                n136 = global read "Global ER2007.vi" "A/D Volts"() -> (w401:dbl[])
              }
              frame True {
                # "Convert to eng units"
                n137 = global read "Global ER2007.vi" "A/D EUs"() -> (w402:dbl[])
              }
            }
            n138 = Array Subset(array=w391, index=0, length=35) -> (w390:dbl[])
            n139 = Index Array(array=w390) -> (element #1=→"Ain 0-0":dbl, element #2=→"Ain 0-1":dbl, element #3=→"Ain 0-2":dbl, element #4=→"Ain 0-3":dbl, element #5=→"Ain 0-8":dbl, element #6=→"Ain 0-9":dbl, element #7=→"Ain 0-10":dbl, element #8=→"Ain 1-0":dbl, element #9=→"Ain 1-1":dbl, element #10=→"Ain 1-2":dbl, element #11=→"Ain 1-3":dbl, element #12=→"Ain 1-5":dbl, element #13=→"Ain 1-6":dbl, element #14=→"Ain 1-7":dbl, element #15=→"Ain 1-8":dbl, element #16=→"Ain 1-9":dbl, element #17=→"Ain 1-10":dbl, element #18=→"Ain 1-11":dbl, element #19=→"Ain 1-13":dbl, element #20=→"Ain 1-14":dbl, element #21=→"Ain 1-15":dbl, element #22=→"Ain 1-16":dbl, element #23=→"Ain 1-17":dbl, element #24=→"Ain 1-18":dbl, element #25=→"Ain 1-19":dbl, element #26=→"Ain 1-21":dbl, element #27=→"Ain 1-22":dbl, element #28=→"Ain 1-23":dbl, element #29=→"Ain 1-24":dbl, element #30=→"Ain 1-25":dbl, element #31=→"Ain 1-26":dbl, element #32=→"Ain 1-27":dbl, element #33=→"Ain 1-29":dbl, element #34=→"Ain 1-30":dbl, element #35=→"Ain 1-31":dbl)  [unwired: 35 in]
            n140 = global read "Global ER2007.vi" "A/D Err"() -> (→"Err 5":bool)
          }
          frame #5 {
            # "Galil CDS-3310"
            n141 = case shown="False" "EUs 1" {
              tunnel: [w419 w420] -> w405
              frame False {
                # "Volts"
                n142 = global read "Global ER2007.vi" "A/D Volts"() -> (w419:dbl[])
              }
              frame True {
                # "Convert to eng units"
                n143 = global read "Global ER2007.vi" "A/D EUs"() -> (w420:dbl[])
              }
            }
            n144 = Array Subset(array=w405, index=35, length=10) -> (w406:dbl[])
            n145 = Index Array(array=w406) -> (element #1=→"Net 0-0":dbl, element #2=→"Net 0-1":dbl, element #3=→"Net 1-0":dbl, element #4=→"Net 1-1":dbl, element #5=→"Net 2-0":dbl, element #6=→"Net 2-1":dbl, element #7=→"Net 3-0":dbl, element #8=→"Net 3-1":dbl, element #9=→"Net 4-0":dbl, element #10=→"Net 4-1":dbl)  [unwired: 10 in]
            n146 = global read "Global ER2007.vi" "Galil Err"() -> (→"Err 6":bool)
          }
          frame #6 {
            # "Agilent 33220A\nFrequency Gen"
            n147 = case shown="False" w429 {
              tunnel: w428 -> [w433 _]
              tunnel: w427 -> [w437 _]
              tunnel: w426 -> [w436 w480]
              tunnel: [w435 w480] -> w425
              tunnel: [w434 w479] -> w424
              tunnel: w423 -> [w430 w479]
              tunnel: w422 -> [w432 _]
              tunnel: [w431 FALSE ("Gen Off/On")] -> w421
              frame False {
                n148 = case shown="False" w437 {
                  tunnel: w436 -> [w438 w477]
                  tunnel: [w443 w464] -> w435
                  tunnel: [w444 w467] -> w434
                  tunnel: w433 -> [_ w473]
                  tunnel: w432 -> [w447 w466]
                  tunnel: [w445 w466] -> w431
                  tunnel: w430 -> [w442 _]
                  frame False {
                    n149 = Not Equal?(x="Gen Off/On", y=w447) -> (x != y?=w441:bool)
                    n150 = Or(x=w441, y="Set") -> (x .or. y?=w440:bool)
                    n151 = case shown="False" w440 {
                      tunnel: w447 -> [w451 _]
                      tunnel: "Gen Off/On" -> [_ w454]
                      tunnel: [w451 w454] -> w445
                      tunnel: [w450 w455] -> w444
                      tunnel: [w448 w452] -> w443
                      tunnel: w442 -> [w450 w462]
                      tunnel: w438 -> [w448 w463]
                      frame False {
                        n152 = Unbundle By Name(w448) -> ("status"=→"Err 3":bool)
                      }
                      frame True {
                        w458 = u16 1 items=["Vpp", "Vrms", "dB"] ("Unit (0: Vpp)")
                        w461 = u16 1 items=["DC"=0, "Sine"=1, "Square"=2, "Triangle"=3, "Ramp"=4, "Pulse"=6, "Noise"=7, "Sinc"=8, "Neg. Ramp"=9, "Exp. Rise"=10, "Exp. Fall"=11, "Cardiac"=12, "Volatile"=13, "User Def. Wfm"=14] ("Waveform Shape (1: Sine)")
                        n153 = call "ag33xxx - Config Waveform.vi"("VISA session"=w462, "Waveform Shape (1: Sine)"=w461, "Frequency (1000 Hz)"="Freq (Hz)", "Amplitude (0.1 Vpp)"="Ampl (Vrms)", "error in (no error)"=w463, "Unit (0: Vpp)"=w458) -> ("dup VISA session"=w457:refnum<visa-resource-name>, "error out"=w456:errorcluster)  [unwired: 8 in]
                        n154 = call "ag33xxx - Output Enabled.vi"("error in (no error)"=w456, "Output Enabled? (T: Yes)"=w454, "VISA session"=w457) -> ("error out"=w453:errorcluster, "dup VISA session"=w455:refnum<visa-resource-name>)  [unwired: 7 in]
                        n155 = call <vilib>:"Simple Error Handler.vi"("error in (no error)"=w453) -> ("error out"=w452:errorcluster)  [unwired: 4 in, 4 out]
                      }
                    }
                  }
                  frame True {
                    w470 = TRUE  # Reset (T: Reset)
                    # "Initialize"
                    n156 = Concatenate Strings("GPIB::" ("string"), w473, "::INSTR" ("string")) -> (w472:string)
                    n157 = Type Cast(type=refnum<visa-resource-name> "GPIB::10::INSTR" ("Instrument Resource Name"), x=w472) -> (*(type *) &x=w471:refnum<visa-resource-name>)
                    n158 = call "ag33xxx - Initialize.vi"("error in (no error)"=w477, "Reset (T: Reset)"=w470, "Instrument Resource Name"=w471) -> ("error out"=w469:errorcluster, "dup VISA session"=w468:refnum<visa-resource-name>)  [unwired: 7 in]
                    n159 = local write "Gen Off/On"(w466) -> ()
                    n160 = call "ag33xxx - Output Enabled.vi"("error in (no error)"=w469, "Output Enabled? (T: Yes)"=w466, "VISA session"=w468) -> ("error out"=w465:errorcluster, "dup VISA session"=w467:refnum<visa-resource-name>)  [unwired: 7 in]
                    n161 = call <vilib>:"Simple Error Handler.vi"("error in (no error)"=w465) -> ("error out"=w464:errorcluster)  [unwired: 4 in, 4 out]
                  }
                }
              }
              frame True {
                # "Simulation"
              }
            }
          }
          frame #7 {
            # "NAII VI's Used:\n1 - NAI2250 Initialize.vi\n2 - NAI2250 Configure.vi\n3 - NAI2250 Measurement Mode.vi\n4 - NAI2250 Measurement Channel.vi\n5 - NAI2250 Measure (Main).vi\n6 - NAI2250 Measure (Select Channel).vi"
            # "Notes\n1- Error code -1074118636 is an \"Out-of-lock frequency condition\".  Use the\n    \"NAI2250 Error Message.vi\" to decipher negative error codes."
            # "Voltage and Phase\nfrom North Atlantic\n2250 DAV"
            n162 = case shown="False" w488 {
              tunnel: w487 -> [w496 w626]
              tunnel: [w492 w626] -> w486
              tunnel: w485 -> [w495 _]
              tunnel: w484 -> [w494 _]
              tunnel: [w491 w625] -> w483
              tunnel: w482 -> [w493 w625]
              tunnel: "Update" -> [w490 w624]
              frame False {
                n163 = case shown="False" w495 {
                  tunnel: w496 -> [w500 _]
                  tunnel: w494 -> [_ w622]
                  tunnel: [w498 w614] -> w492
                  tunnel: w493 -> [w501 _]
                  tunnel: [w499 w615] -> w491
                  tunnel: w490 -> [w497 _]
                  frame False {
                    n164 = case shown="True" w497 {
                      tunnel: w501 -> [w504 w508]
                      tunnel: w500 -> [w502 w506]
                      tunnel: [w504 w507] -> w499
                      tunnel: [w502 w505] -> w498
                      frame False {
                        n165 = Unbundle By Name(w502) -> ("status"=→"Err 4":bool)
                      }
                      frame True {
                        n166 = stacked-sequence {
                          seq-local: [_ w511 _ _ _ _ _ _ _ _ _] -> [_ _ w520 _ _ _ _ _ _ _ _]
                          seq-local: [_ _ _ _ w538 _ _ _ _ _ _] -> [_ _ _ _ _ _ _ _ _ _ _]
                          seq-local: [_ _ _ _ _ w552 _ _ _ _ _] -> [_ _ _ _ _ _ w562 _ _ _ _]
                          seq-local: [_ _ w518 _ _ _ _ _ _ _ _] -> [_ _ _ w536 _ _ _ _ _ _ _]
                          seq-local: [_ _ _ w532 _ _ _ _ _ _ _] -> [_ _ _ _ w543 _ _ _ _ _ _]
                          seq-local: [_ _ _ _ _ _ w558 _ _ _ _] -> [_ _ _ _ _ _ _ w575 _ _ _]
                          seq-local: [_ "Wait (ms)" _ _ _ _ _ _ _ _ _] -> [_ _ w519 _ w539 _ w557 _ w577 w591 _]
                          seq-local: [_ _ _ _ _ _ _ w570 _ _ _] -> [_ _ _ _ _ _ _ _ w579 _ _]
                          seq-local: [_ _ _ _ _ _ _ _ w576 _ _] -> [_ _ _ _ _ _ _ _ _ w594 _]
                          seq-local: [w509 _ _ _ _ _ _ _ _ _ _] -> [_ _ _ _ _ _ _ _ _ _ w612]
                          tunnel: w508 -> [_ w516 w521 w537 w540 w556 w559 w574 w578 w589 _]
                          tunnel: [_ _ _ _ _ _ _ _ _ w589 _] -> w507
                          tunnel: w506 -> [_ w515 _ _ _ _ _ _ _ _ _]
                          tunnel: [_ _ _ _ _ _ _ _ _ w595 _] -> w505
                          frame #0 {
                            n167 = Tick Count (ms)() -> (millisecond timer value=w509:u32)
                          }
                          frame #1 {
                            w510 = TRUE  # Reference
                            # "NAI2250 Measurement Channel.vi"
                            # "NAI2250 Measurement Mode.vi"
                            # "Requests Reference voltage"
                            n168 = call "AC2250 Measurement Mode.vi"("ErrIn"=w515, "Measurement Mode"=T1."TOTAL", "VISA Resource Name In"=w516) -> ("ErrOut"=w512:errorcluster, "VISA Resource Name Out"=w513:refnum<visa-resource-name>)  [unwired: 6 in, 1 out]
                            n169 = call "AC2250 Measurement Channel.vi"("ErrIn"=w512, "Reference"=w510, "VISA Resource Name In"=w513) -> ("ErrOut"=w511:errorcluster)  [unwired: 6 in, 2 out]
                          }
                          frame #2 {
                            # "Reads\nReference\nVoltage"
                            n170 = flat-sequence {
                              tunnel: w520 -> [w526]
                              tunnel: [w526] -> w523
                              tunnel: w521 -> [w525]
                              tunnel: [w525] -> w522
                              tunnel: w519 -> [w524]
                              tunnel: w523 -> [w528]
                              tunnel: [w530] -> w518
                              tunnel: w522 -> [w529]
                              frame #0 {
                                # "Waits"
                                n171 = Wait (ms)(milliseconds to wait=w524) -> ()  [unwired: 1 out]
                              }
                              frame #1 {
                                # "NAI2250 Measure (Main).vi"
                                n172 = call "AC2250 Measure (Main).vi"("ErrIn"=w528, "VISA Resource Name In"=w529) -> ("ErrOut"=w530:errorcluster, "Value"=→"Reference":dbl)  [unwired: 5 in, 3 out]
                              }
                            }
                          }
                          frame #3 {
                            w531 = FALSE  # Reference
                            # "NAI2250 Measurement Channel.vi"
                            # "NAI2250 Measurement Mode.vi"
                            # "Requests Signal voltage"
                            n173 = call "AC2250 Measurement Mode.vi"("ErrIn"=w536, "Measurement Mode"=T1."TOTAL", "VISA Resource Name In"=w537) -> ("ErrOut"=w533:errorcluster, "VISA Resource Name Out"=w534:refnum<visa-resource-name>)  [unwired: 6 in, 1 out]
                            n174 = call "AC2250 Measurement Channel.vi"("ErrIn"=w533, "Reference"=w531, "VISA Resource Name In"=w534) -> ("ErrOut"=w532:errorcluster)  [unwired: 6 in, 2 out]
                          }
                          frame #4 {
                            # "Reads\nSignal\nVoltage"
                            n175 = flat-sequence {
                              tunnel: w543 -> [w546]
                              tunnel: [w546] -> w542
                              tunnel: w540 -> [w545]
                              tunnel: [w545] -> w541
                              tunnel: w539 -> [w544]
                              tunnel: w542 -> [w550]
                              tunnel: w541 -> [w547]
                              tunnel: [w549] -> w538
                              frame #0 {
                                # "Waits"
                                n176 = Wait (ms)(milliseconds to wait=w544) -> ()  [unwired: 1 out]
                              }
                              frame #1 {
                                # "NAI2250 Measure (Main).vi"
                                n177 = call "AC2250 Measure (Main).vi"("ErrIn"=w550, "VISA Resource Name In"=w547) -> ("ErrOut"=w549:errorcluster, "Value"=→"Signal":dbl)  [unwired: 5 in, 3 out]
                              }
                            }
                          }
                          frame #5 {
                            w551 = FALSE  # Reference
                            # "NAI2250 Measurement Channel.vi"
                            # "NAI2250 Measurement Mode.vi"
                            # "Requests Signal phase angle"
                            n178 = call "AC2250 Measurement Mode.vi"("Measurement Mode"=T1."PHASE ANGLE", "VISA Resource Name In"=w556) -> ("ErrOut"=w553:errorcluster, "VISA Resource Name Out"=w554:refnum<visa-resource-name>)  [unwired: 7 in, 1 out]
                            n179 = call "AC2250 Measurement Channel.vi"("ErrIn"=w553, "Reference"=w551, "VISA Resource Name In"=w554) -> ("ErrOut"=w552:errorcluster)  [unwired: 6 in, 2 out]
                          }
                          frame #6 {
                            # "Reads Phase angle"
                            n180 = flat-sequence {
                              tunnel: w562 -> [w565]
                              tunnel: [w565] -> w561
                              tunnel: w559 -> [w564]
                              tunnel: [w564] -> w560
                              tunnel: w557 -> [w563]
                              tunnel: w561 -> [w569]
                              tunnel: [w568] -> w558
                              tunnel: w560 -> [w567]
                              frame #0 {
                                # "Waits"
                                n181 = Wait (ms)(milliseconds to wait=w563) -> ()  [unwired: 1 out]
                              }
                              frame #1 {
                                # "NAI2250 Measure (Main).vi"
                                n182 = call "AC2250 Measure (Main).vi"("ErrIn"=w569, "VISA Resource Name In"=w567) -> ("ErrOut"=w568:errorcluster, "Value"=→"Phase":dbl)  [unwired: 5 in, 3 out]
                              }
                            }
                          }
                          frame #7 {
                            # "Requests Signal frequency"
                            n183 = Concatenate Strings("INX FREQ" ("write buffer"), "\r\n") -> (w573:string)
                            n184 = VISA Write(VISA resource name=w574, write buffer=w573, error in (no error)=w575) -> (error out=w570:errorcluster)  [unwired: 2 out]
                          }
                          frame #8 {
                            n185 = flat-sequence {
                              tunnel: w579 -> [w584]
                              tunnel: [w584] -> w581
                              tunnel: w578 -> [w583]
                              tunnel: [w583] -> w580
                              tunnel: w577 -> [w582]
                              tunnel: w581 -> [w588]
                              tunnel: [w585] -> w576
                              tunnel: w580 -> [w587]
                              frame #0 {
                                # "Waits"
                                n186 = Wait (ms)(milliseconds to wait=w582) -> ()  [unwired: 1 out]
                              }
                              frame #1 {
                                # "was NAI2250 Measure (Select Channel).vi"
                                # "Reads frequency"
                                n187 = call "AC2250 Measure (Main).vi"("ErrIn"=w588, "VISA Resource Name In"=w587) -> ("ErrOut"=w585:errorcluster, "Value"=→"Freq":dbl)  [unwired: 5 in, 3 out]
                              }
                            }
                          }
                          frame #9 {
                            # "Reports errors, resets latch"
                            n188 = flat-sequence {
                              tunnel: w594 -> [w599]
                              tunnel: [w599] -> w592
                              tunnel: w591 -> [w598]
                              tunnel: w589 -> [w597]
                              tunnel: [w597] -> w590
                              tunnel: [w601] -> w593
                              tunnel: w592 -> [w602]
                              tunnel: w590 -> [w600]
                              tunnel: [w606] -> w596
                              tunnel: w593 -> [w607]
                              tunnel: w596 -> [w609]
                              tunnel: [w609] -> w595
                              frame #0 {
                                n189 = Wait (ms)(milliseconds to wait=w598) -> ()  [unwired: 1 out]
                              }
                              frame #1 {
                                n190 = Concatenate Strings("INX MAIN" ("write buffer"), "\r\n") -> (w603:string)
                                n191 = VISA Write(VISA resource name=w600, write buffer=w603, error in (no error)=w602) -> (error out=w601:errorcluster)  [unwired: 2 out]
                              }
                              frame #2 {
                                n192 = Unbundle By Name(w607) -> ("code"=→"NAII Err":i32)
                                n193 = call <vilib>:"Simple Error Handler.vi"("error in (no error)"=w607) -> ("error out"=w606:errorcluster)  [unwired: 4 in, 4 out]
                              }
                              frame #3 {
                                n194 = local write "Update"(FALSE ("Update")) -> ()
                              }
                            }
                          }
                          frame #10 {
                            n195 = Tick Count (ms)() -> (millisecond timer value=w613:u32)
                            n196 = Subtract(x=w613, y=w612) -> (x-y=→"NAII Time":u32)
                          }
                        }
                      }
                    }
                  }
                  frame True {
                    w623 = 0.0 ("Reference")
                    # "NAI2250 Configure.vi"
                    # "NAI2250 Initialize.vi"
                    # "Initialize"
                    n197 = Concatenate Strings("GPIB::" ("string"), w622, "::INSTR" ("string")) -> (w619:string)
                    n198 = call "AC2250 Initialize.vi"("VISA Resource Name In"=w619) -> ("ErrOut"=w617:errorcluster, "VISA Resource Name Out"=w618:refnum<visa-resource-name>)  [unwired: 9 in]
                    n199 = call "AC2250 Configure.vi"("ErrIn"=w617, "Measurement Mode"=T1."TOTAL", "VISA Resource Name In"=w618) -> ("ErrOut"=w614:errorcluster, "VISA Resource Name Out"=w615:refnum<visa-resource-name>)  [unwired: 6 in, 1 out]
                    n200 = local write "Reference"(w623) -> ()
                    n201 = call <vilib>:"Simple Error Handler.vi"("error in (no error)"=w614) -> ()  [unwired: 4 in, 5 out]
                    n202 = local write "Signal"(w623) -> ()
                    n203 = local write "Phase"(w623) -> ()
                  }
                }
              }
              frame True {
                # "Simulation"
                n204 = case shown="True" w624 {
                  frame False {
                  }
                  frame True {
                    n205 = local write "Update"(FALSE ("Update")) -> ()
                  }
                }
              }
            }
          }
          frame #8 {
            n206 = Tick Count (ms)() -> (millisecond timer value=w630:u32)
            n207 = Subtract(x=w630, y=w629) -> (x-y=→"Exec Time":u32)
          }
        }
        n208 = Wait Until Next ms Multiple(millisecond multiple=u32 333) -> ()  [unwired: 1 out]
      }
    }
    frame #2 {
      # "SimHP"
      # "SimNAI"
      # "SimDAQ"
      # "SysRun"
      # "Cleanup and shutdown"
      n209 = stacked-sequence {
        tunnel: w640 -> [_ _ w675 _]
        tunnel: w639 -> [_ _ w674 _]
        tunnel: w638 -> [_ w655 w673 w683]
        tunnel: w637 -> [w650 _ _ _]
        tunnel: w636 -> [w649 _ _ _]
        tunnel: w635 -> [w646 _ _ _]
        tunnel: w634 -> [w645 _ _ _]
        tunnel: w633 -> [w644 _ _ _]
        tunnel: w632 -> [w642 _ _ _]
        tunnel: w631 -> [w643 _ _ _]
        frame #0 {
          w648 = FALSE ("Visible")
          w647 = FALSE ("Err 1")
          # "Closes all I/O tasks"
          n210 = property on="Exec Time" class="DigNum (strict)"("Visible"=w648) -> ()  [unwired: 2 in, 2 out]
          n211 = property on="Dout 0-1.6" class="Bool (strict)"("Disabled"=u8 0) -> ()  [unwired: 2 in, 2 out]
          n212 = local write "Dev1Err"(w647) -> ()
          n213 = property on="NAII Err" class="DigNum (strict)"("Visible"=w648) -> ()  [unwired: 2 in, 2 out]
          n214 = local write "Err 7"(w647) -> ()
          n215 = property on="NAII Time" class="DigNum (strict)"("Visible"=w648) -> ()  [unwired: 2 in, 2 out]
          n216 = local write "Err 5"(w647) -> ()
          n217 = local write "Err 6"(w647) -> ()
          n218 = local write "Err 3"(w647) -> ()
          n219 = local write "Err 4"(w647) -> ()
          n220 = case shown="False" w644 {
            tunnel: w650 -> [w654 _]
            tunnel: w649 -> [w653 _]
            frame False {
              n221 = call <vilib>:"DAQmx Clear Task.vi"("task in"=w654) -> ()  [unwired: 14 in, 1 out]
              n222 = call <vilib>:"DAQmx Clear Task.vi"("task in"=w653) -> ()  [unwired: 14 in, 1 out]
            }
            frame True {
            }
          }
          n223 = case shown="False" w642 {
            tunnel: w645 -> [w651 _]
            frame False {
              n224 = VISA Close(VISA resource name=w651) -> ()  [unwired: 1 in, 1 out]
            }
            frame True {
            }
          }
          n225 = case shown="False" w643 {
            tunnel: w646 -> [w652 _]
            frame False {
              n226 = call "ag33xxx - Close.vi"("VISA session"=w652) -> ()  [unwired: 10 in, 1 out]
            }
            frame True {
            }
          }
        }
        frame #1 {
          n227 = case shown="True" w655 {
            frame False {
            }
            frame True {
              # "SysRun - restarts the Get Cell Data vi"
              n228 = stacked-sequence {
                seq-local: [w657 _] -> [_ w663]
                frame #0 {
                  n229 = global read "Global ER2007.vi" "BckGetEng vi name"() -> (w656:path)
                  n230 = Get Date/Time In Seconds() -> (seconds since 1Jan1904=w658:timestamp)
                  n231 = To Double Precision Float(number=w658) -> (double precision float=w657:dbl)
                  n232 = Open VI Reference(vi path=w656) -> (vi reference=w659:refnum<vi>)  [unwired: 5 in, 1 out]
                  n233 = invoke class="VI" method="Run VI"(reference=w659, "Wait until done"=FALSE, "Auto Dispose Ref"=TRUE) -> (error out=w662:errorcluster)  [unwired: 2 in, 4 out]
                  n234 = call <vilib>:"Simple Error Handler.vi"("error in (no error)"=w662) -> ()  [unwired: 4 in, 5 out]
                }
                frame #1 {
                  n235 = while {
                    tunnel: w663 -> [w670]
                    stop <- w666 stop-if-true
                    # "Waits for Run flag or T/O"
                    n236 = Get Date/Time In Seconds() -> (seconds since 1Jan1904=w672:timestamp)
                    n237 = global read "Global ER2007.vi" "GCD Run"() -> (w664:bool)
                    n238 = To Double Precision Float(number=w672) -> (double precision float=w671:dbl)
                    n239 = Wait Until Next ms Multiple(millisecond multiple=u32 250) -> ()  [unwired: 1 out]
                    n240 = Subtract(x=w671, y=w670) -> (x-y=w669:dbl)
                    n241 = Greater?(x=w669, y=2.0) -> (0:w665:bool)
                    n242 = Or(x=w665, y=w664) -> (x .or. y?=w666:bool)
                  }
                }
              }
            }
          }
        }
        frame #2 {
          # "Opens the Utilities front panel"
          n243 = case shown="False" w673 {
            tunnel: w675 -> [_ w682]
            tunnel: w674 -> [_ w681]
            frame False {
              # "Not a System run"
              n244 = global write "Global ER2007.vi" "DAQ Stop"(TRUE ("A/D Init")) -> ()
            }
            frame True {
              # "System run"
              n245 = property class="VI"(reference=w682, error in=w681, "Front Panel Window:Open"=TRUE) -> (reference out=w679:refnum<vi>, error out=w678:errorcluster)
              n246 = Close Reference(reference=w679, error in (no error)=w678) -> (error out=w677:errorcluster)
              n247 = call <vilib>:"Simple Error Handler.vi"("error in (no error)"=w677) -> ()  [unwired: 4 in, 5 out]
            }
          }
        }
        frame #3 {
          # "Closes this panel"
          n248 = case shown="True" w683 {
            frame False {
            }
            frame True {
              n249 = Current VI's Path() -> (path=w690:path)
              n250 = Open VI Reference(vi path=w690) -> (vi reference=w689:refnum<vi>, error out=w688:errorcluster)  [unwired: 5 in]
              n251 = property class="VI"(reference=w689, error in=w688, "Front Panel Window:Open"=FALSE) -> (reference out=w686:refnum<vi>, error out=w685:errorcluster)
              n252 = Close Reference(reference=w686, error in (no error)=w685) -> (error out=w684:errorcluster)
              n253 = call <vilib>:"Simple Error Handler.vi"("error in (no error)"=w684) -> ()  [unwired: 4 in, 5 out]
            }
          }
        }
      }
    }
  }
